vi "thcd_set_dsp.vi"(5 "thcd_delay":u32=500, 6 "err_in":errorcluster, 7 "thcd_val":T1, 8 "thcd_ch":T2, 9 "thcd_visa":refnum<visa-resource-name>) -> (0 "err_out":errorcluster, 1 "thcd_st":bool, 2 "thcd_res_msg":string, 3 "thcd_visa":refnum<visa-resource-name>)   [LabVIEW 2019]
uses:
  thcd_controls/ctrl_chn_thcd.ctl
  thcd_controls/ctrl_dsp_thcd.ctl
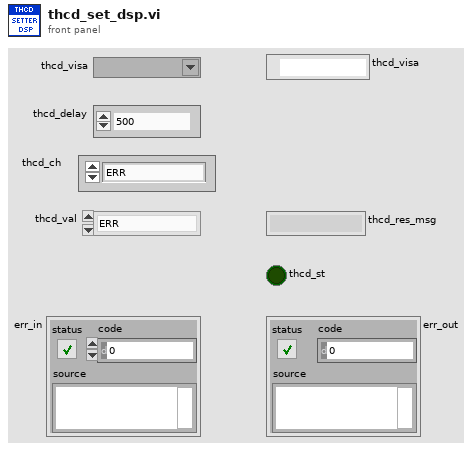
[diagram p1: front panel]
types:
  T1 = typedef "ctrl_dsp_thcd.ctl" = enum16{"ERR", "TOTAL", "FLOW", "BLANK"}
  T2 = typedef "ctrl_chn_thcd.ctl" = enum8{"ERR", "1", "2", "3", "4"}
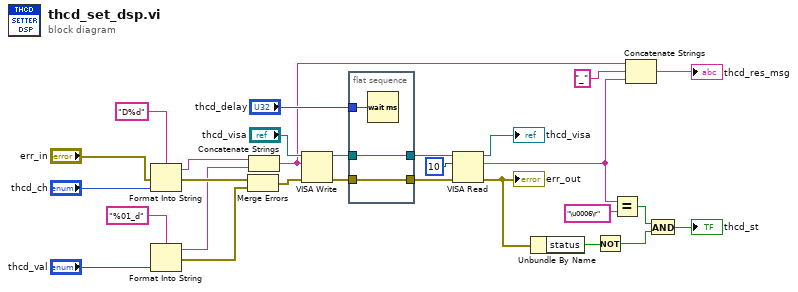
[diagram p0: block diagram]
diagram:
  n1 = Format Into String(format string="D%d", error in="err_in", "thcd_ch") -> (resulting string=w18:string, error out=w17:errorcluster)  [unwired: 1 in]
  n2 = Format Into String(format string="%01_d", "thcd_val") -> (resulting string=w14:string, error out=w15:errorcluster)  [unwired: 2 in]
  n3 = Merge Errors(w17, w15) -> (w16:errorcluster)
  n4 = Concatenate Strings(w18, w14) -> (w1:string)
  n5 = VISA Write(VISA resource name="thcd_visa", write buffer=w1, error in (no error)=w16) -> (VISA resource name out=w26:refnum<visa-resource-name>, error out=w27:errorcluster)  [unwired: 1 out]
  n6 = flat-sequence {
    tunnel: w27 -> [w29]
    tunnel: [w29] -> w5
    tunnel: w26 -> [w28]
    tunnel: [w28] -> w7
    tunnel: "thcd_delay" -> [w30]
    frame #0 {
      n7 = Wait (ms)(milliseconds to wait=w30) -> ()  [unwired: 1 out]
    }
  }
  n8 = VISA Read(VISA resource name=w7, byte count=u32 10) -> (VISA resource name out=→"thcd_visa":refnum<visa-resource-name>, read buffer=w8:string)  [unwired: 1 in, 2 out]
  n9 = Unbundle By Name(w5) -> ("status"=w19:bool)
  n10 = Not(x=w19) -> (.not. x?=w4:bool)
  n11 = Equal?(x=w8, y="\u0006\r") -> (x = y?=w11:bool)
  n12 = Concatenate Strings(w1, "_", w8) -> (→"thcd_res_msg":string)
  n13 = And(x=w11, y=w4) -> (x .and. y?=→"thcd_st":bool)
  "err_out" <- w5
